vi "Configure UCP State and Level.vi"(6 "UCP Warm(S)":dbl min=0.0 max=30.0, 7 "State":bool, 8 "error in":errorcluster, 9 "UCP Delay(S)":dbl min=0.0 max=10.0, 10 "UCP Level(A)":dbl min=0.0 max=3.5, 11 "VISA resource name":refnum<visa-resource-name>) -> (0 "error out":errorcluster, 3 "VISA resource name out":refnum<visa-resource-name>)   [LabVIEW 2018, in "IT-M3100.lvlib"]
doc: "This command enables or disables the under-current function.\n<b>State</b>\n0:Close the State\n1:Open the state\n<b>UCP Level(A)</b>\n0-3.5\n<b>UCP Delay(S)</b>\n0-10\n<b>UCP Warm(S)</b>\n0-30"
uses:
  IT-M3100.lvlib
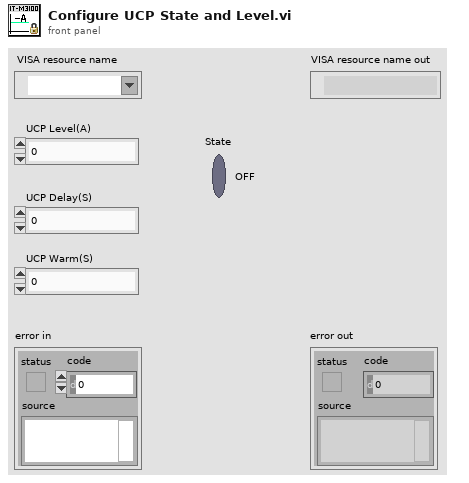
[diagram p1: front panel]
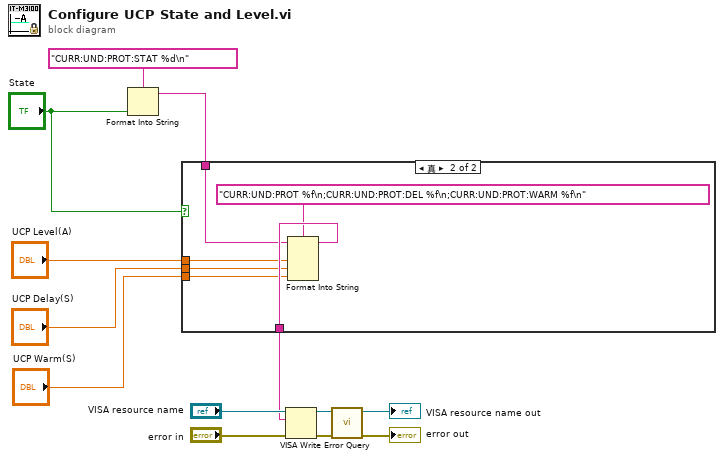
[diagram p0: block diagram]
diagram:
  n1 = Format Into String(format string="CURR:UND:PROT:STAT %d\n", "State") -> (resulting string=w5:string)  [unwired: 2 in, 1 out]
  n2 = case shown="真" "State" {
    tunnel: w5 -> [w14 w18]
    tunnel: [w14 w20] -> w6
    tunnel: "UCP Level(A)" -> [_ w17]
    tunnel: "UCP Delay(S)" -> [_ w16]
    tunnel: "UCP Warm(S)" -> [_ w15]
    frame False {
    }
    frame True {
      n3 = Format Into String(format string="CURR:UND:PROT %f\n;CURR:UND:PROT:DEL %f\n;CURR:UND:PROT:WARM %f\n", initial string=w18, w17, w16, w15) -> (resulting string=w20:string)  [unwired: 1 in, 1 out]
    }
  }
  n4 = VISA Write(VISA resource name="VISA resource name", write buffer=w6, error in (no error)="error in") -> (VISA resource name out=w10:refnum<visa-resource-name>, error out=w11:errorcluster)  [unwired: 1 out]
  n5 = call "Error Query.vi"("error in"=w11, "VISA resource name"=w10) -> ("error out"=→"error out":errorcluster, "VISA resource name out"=→"VISA resource name out":refnum<visa-resource-name>)  [unwired: 6 in, 2 out]
